vi "Initialize MeasurementLink Session.vi"(7 "remote connection options":T2, 8 "error in":errorcluster, 9 "initialize and close session behavior":T1, 10 "session initialization parameters":T3, 11 "KeysightDmm in":refnum<class "KeysightDmm.lvclass">) -> (0 "error out":errorcluster, 2 "session out":variant, 3 "KeysightDmm out":refnum<class "KeysightDmm.lvclass">)   [LabVIEW 2021, in "KeysightDmm.lvclass"]
doc: "Creates a new session using the provided <b>session initialization parameters</b>. If the session represents a remote session, <b>initialize and close session behavior</b> determines whether creating the local session creates a new session on the server or attaches to an existing session on the server."
uses:
  KeysightDmm.lvclass
  <vilib>/Plug-In SDKs/Sessions/Instrument/ISession Factory/Session Initialization Parameters.ctl
  <vilib>/Plug-In SDKs/Sessions/Instrument/ISession Factory/Remote Connection Options.ctl
  <vilib>/Plug-In SDKs/Sessions/Instrument/ISession Factory/Initialize and Close Session Behavior.ctl
  KeysightDmm.lvclass/KeysightDmm.ctl
  <vilib>/Plug-In SDKs/Sessions/Instrument/ISession Factory/ISession Factory.lvclass
  <instrlib>/Agilent 34401/Public/Initialize.vi
  <instrlib>/Agilent 34401/Agilent 34401.lvlib
  <vilib>/NI-VISA/VISA Open for gRPC Session.vi
  subVIs/Get VISA gRPC Open Close Behavior.vi
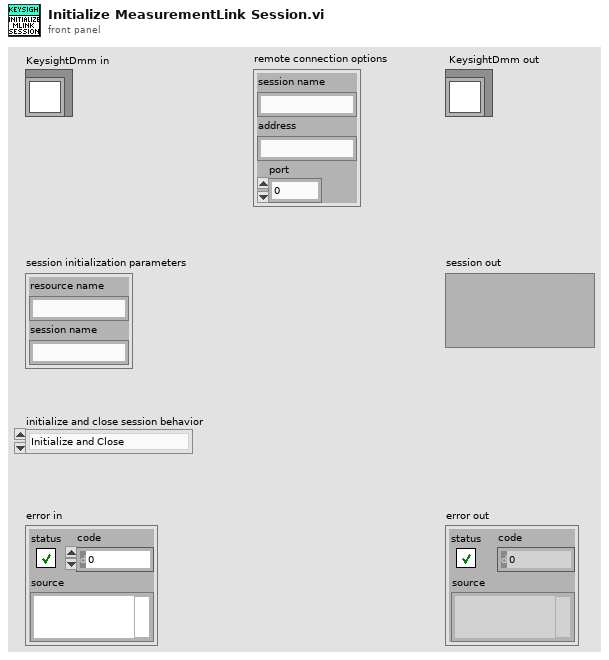
[diagram p1: front panel]
types:
  T1 = typedef "NI Session Management Instrument.lvlib/ISession Factory.lvclass/Initialize and Close Session Behavior.ctl" = enum16{"Initialize and Close", "Attach and Detach", "Initialize and Detach", "Attach and Close"}
  T2 = typedef "NI Session Management Instrument.lvlib/ISession Factory.lvclass/Remote Connection Options.ctl" = cluster{"session name":string, "address":string, "port":u32}
  T3 = typedef "NI Session Management Instrument.lvlib/ISession Factory.lvclass/Session Initialization Parameters.ctl" = cluster{"resource name":string, "session name":string}
  T4 = typedef "VISA gRPC Open Close Behavior.ctl" = enum16{"Auto", "Initialize and Close", "Attach and Detach", "Initialize and Detach", "Attach and Close"}
  T5 = cluster{"Baud Rate":u32, "Parity":u16, "Data Bits":u16}
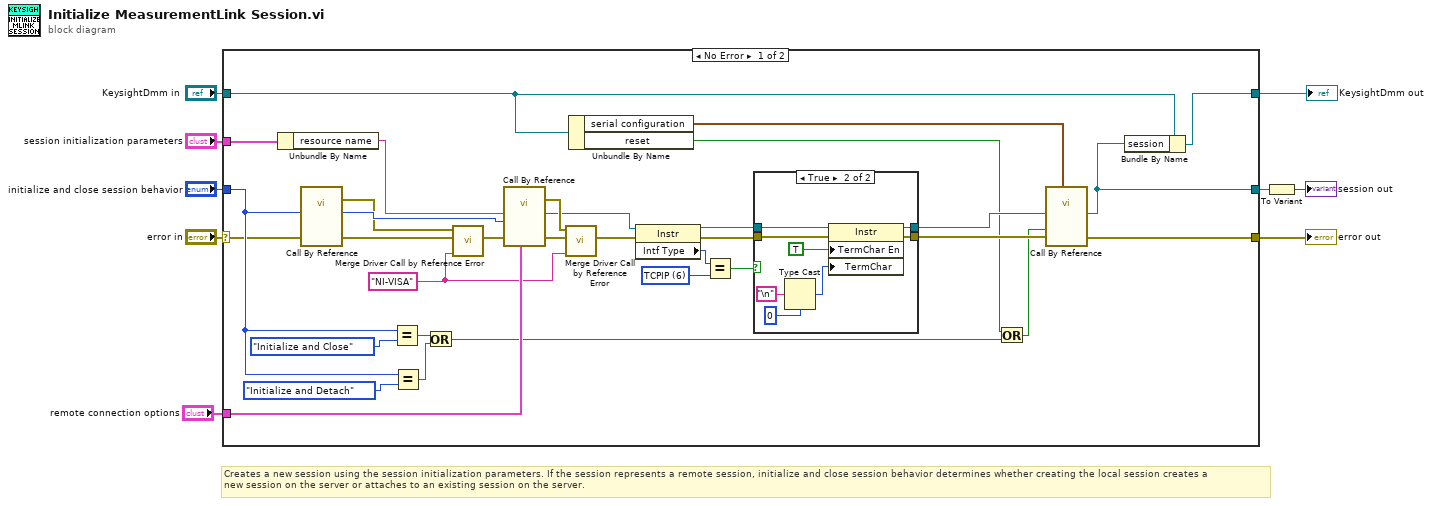
[diagram p0: block diagram]
diagram:
  # "Creates a new session using the session initialization parameters. If the session represents a remote session, initialize and close session behavior determines whether creating the local session creates a \nnew session on the server or attaches to an existing session on the server."
  n1 = case shown="No Error" "error in" {
    selector: "error in" -> [w13 w53]
    tunnel: [w18 w53] -> w9
    tunnel: "KeysightDmm in" -> [w15 w54]
    tunnel: "initialize and close session behavior" -> [w14 _]
    tunnel: "remote connection options" -> [w37 _]
    tunnel: [w16 w54] -> w4
    tunnel: [w17 _] -> w3
    tunnel: "session initialization parameters" -> [w36 _]
    frame No Error {
      w29 = u16 6 items=["GPIB"=1, "VXI"=2, "GPIB-VXI"=3, "Serial"=4, "PXI"=5, "TCPIP"=6, "USB"=7, "FireWire"=9] ("Interface Information:Interface Type")
      w32 = "NI-VISA" ("driver name")
      n2 = Unbundle By Name(w36) -> ("resource name"=w35:string)
      n3 = call-by-ref "?"("initialize session behavior"=w14, "error in (no error)"=w13) -> (error out=w11:errorcluster, "open/close behavior"=w12:T4, 15:"error out"=w10:errorcluster)  [unwired: 14 in, 1 out]
      n4 = Equal?(x=w14, y=Initialize_and_Close_Session_Behavior."Initialize and Close" ("initialize session behavior")) -> (x = y?=w40:bool)
      n5 = Equal?(x=w14, y=Initialize_and_Close_Session_Behavior."Initialize and Detach" ("initialize session behavior")) -> (x = y?=w39:bool)
      n6 = Or(x=w40, y=w39) -> (x .or. y?=w21:bool)
      n7 = call <vilib>:"Merge Driver Call by Reference Error.vi"("driver name"=w32, "called vi error"=w10, "call by ref error"=w11) -> ("error out"=w38:errorcluster)  [unwired: 8 in]
      n8 = call-by-ref "?"("gRPC Options"=w37, "error in (no error)"=w38, "Open/Close Behavior"=w12, "VISA resource name"=w35) -> (error out=w33:errorcluster, 0:"error out"=w34:errorcluster, "VISA resource name out"=w24:refnum<visa-resource-name>)  [unwired: 8 in, 1 out]
      n9 = call <vilib>:"Merge Driver Call by Reference Error.vi"("driver name"=w32, "called vi error"=w34, "call by ref error"=w33) -> ("error out"=w27:errorcluster)  [unwired: 8 in]
      n10 = Unbundle By Name(w15) -> ("serial configuration"=w22:T5, "reset"=w19:bool)
      n11 = property class="Instr"(reference=w24, error in=w27) -> (reference out=w25:refnum<visa-resource-name>, error out=w26:errorcluster, "Intf Type"=w28:u16)
      n12 = Equal?(x=w28, y=w29) -> (x = y?=w23:bool)
      n13 = case shown="True" w23 {
        tunnel: w26 -> [w44 w52]
        tunnel: [w44 w51] -> w31
        tunnel: w25 -> [w43 w50]
        tunnel: [w43 w49] -> w30
        frame False {
        }
        frame True {
          n14 = Type Cast(type=u8 0, x="\n" ("Line Feed Constant")) -> (*(type *) &x=w45:u8)
          n15 = property class="Instr"(reference=w50, error in=w52, "TermChar En"=TRUE ("Message Based Settings:Termination Character Enable"), "TermChar"=w45) -> (reference out=w49:refnum<visa-resource-name>, error out=w51:errorcluster)
        }
      }
      n16 = Or(x=w19, y=w21) -> (x .or. y?=w20:bool)
      n17 = call-by-ref "?"("Serial Configuration"=w22, "error in (no error)"=w31, "Reset (True)"=w20, "VISA resource name"=w30) -> ("error out"=w18:errorcluster, "VISA resource name out"=w17:refnum<visa-resource-name>)  [unwired: 8 in, 2 out]
      n18 = Bundle By Name(cluster=w15, "session"=w17) -> (w16:refnum<class "KeysightDmm.lvclass">)
    }
    frame Error {
    }
  }
  "error out" <- w9
  "KeysightDmm out" <- w4
  n19 = To Variant(anything=w3) -> (Variant=→"session out":variant)
